vi "sync.destroy.vi"(8 "error in (no error)":errorcluster, 11 "synchronization":refnum<class "synchronization.lvclass">) -> (0 "error out":errorcluster)   [LabVIEW 2020, in "synchronization.lvclass"]
uses:
  synchronization.lvclass
  synchronization.lvclass/synchronization.ctl
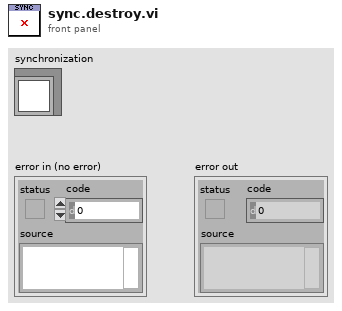
[diagram p1: front panel]
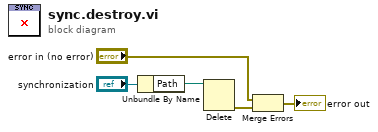
[diagram p0: block diagram]
diagram:
  n1 = Unbundle By Name("synchronization") -> ("Path"=w4:path)
  n2 = Delete(path (use dialog)=w4) -> (error out=w2:errorcluster)  [unwired: 4 in, 2 out]
  n3 = Merge Errors("error in (no error)", w2) -> (→"error out":errorcluster)
